vi "Edit Time Entry.vi"(8 "error in (no error)":errorcluster, 10 "Projects.lvclass":refnum<class "Projects.lvclass">, 11 "Time Entries in":refnum<class "Time Entries.lvclass">) -> (0 "error out":errorcluster, 3 "Time Entries out":refnum<class "Time Entries.lvclass">)   [LabVIEW 2020, in "Time Entries.lvclass"]
doc: "UI to edit the editable properties of the time entry.\n\n08/2025 Erich Schlieper"
uses:
  Time Entries.lvclass
  Projects/Parent/Projects.lvclass
  Time Entries.lvclass/Time Entries.ctl
panel:
  in  "Task":u16(ring)
  in  "Project":u16(ring)
  in  "End Time":timestamp format="%<%x %.3X>T"
  in  "Start Time":timestamp format="%<%x %.3X>T"
  in  "Description":string
  in  "Cancel":bool
  in  "OK":bool
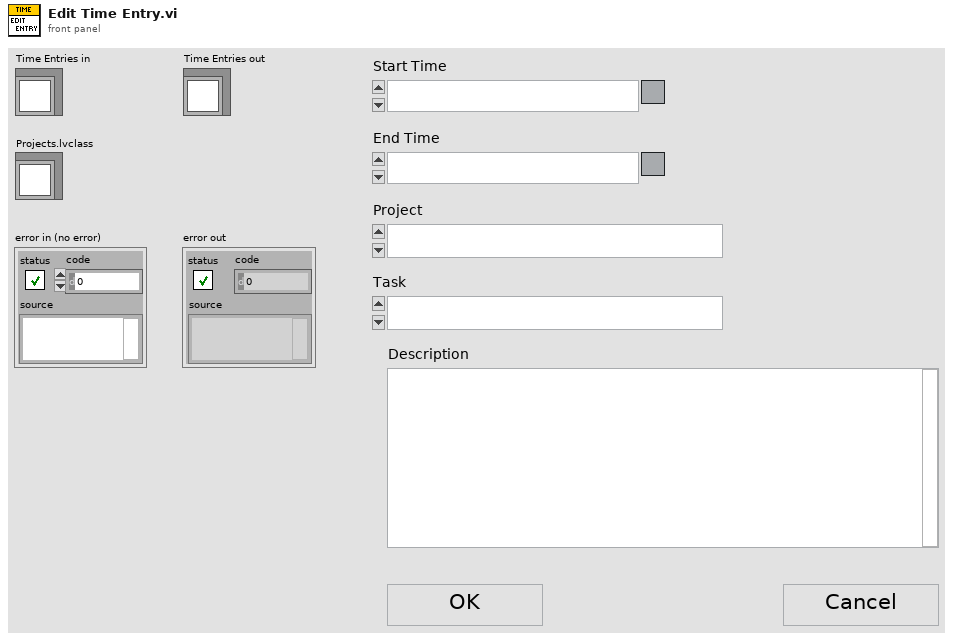
[diagram p1: front panel]
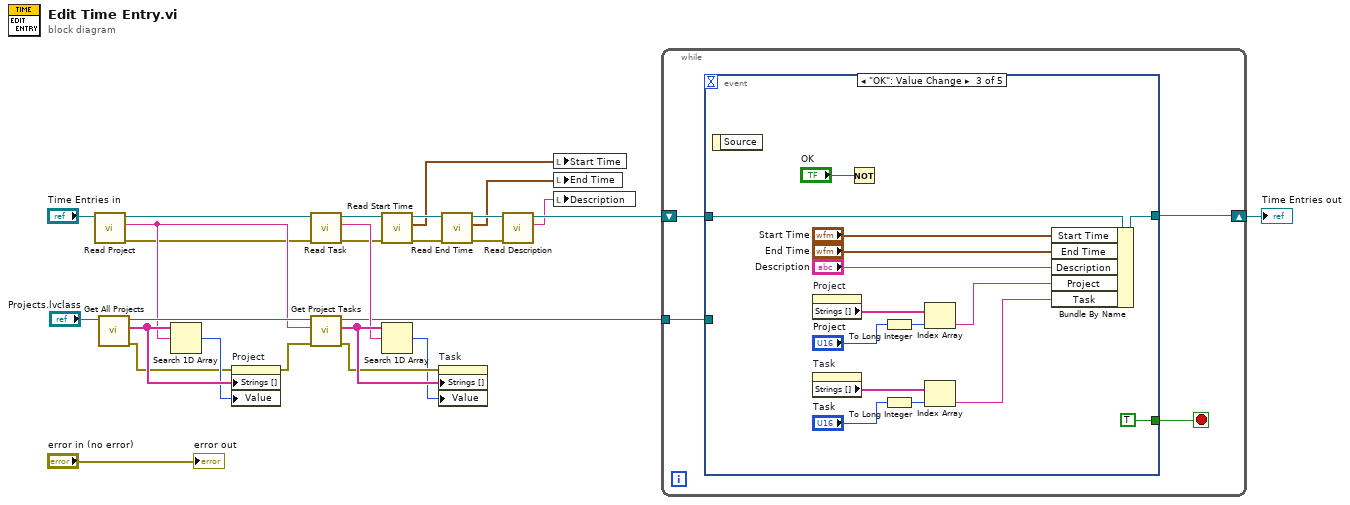
[diagram p0: block diagram]
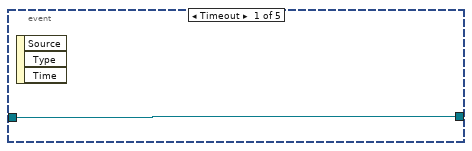
[diagram p2: hidden frame]
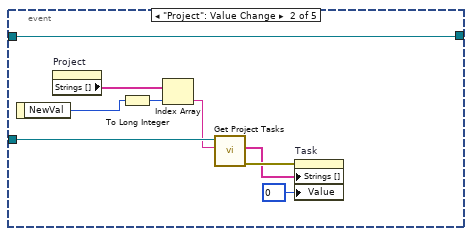
[diagram p3: hidden frame]
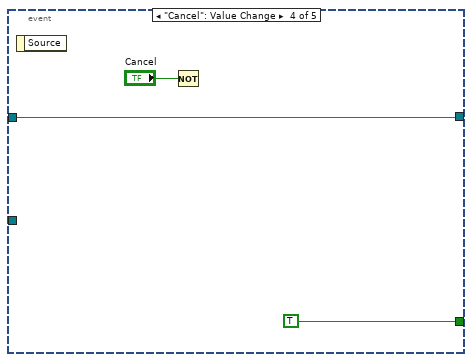
[diagram p4: hidden frame]
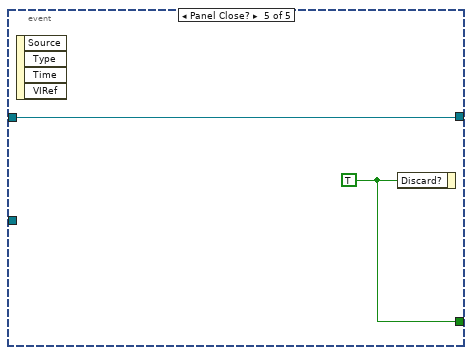
[diagram p5: hidden frame]
diagram:
  n1 = call-dynamic "Read Project.vi"("Time Entries in"="Time Entries in") -> ("error out"=w14:errorcluster, "Project"=w23:string, "Time Entries out"=w19:refnum<class "Time Entries.lvclass">)  [unwired: 8 in]
  n2 = call-dynamic "Get All Projects.vi"("Projects in"="Projects.lvclass") -> ("error out"=w21:errorcluster, "Projects"=w24:string[], "Projects out"=w25:refnum<class "Projects.lvclass">)  [unwired: 8 in]
  n3 = Search 1D Array(1D array=w24, element=w23) -> (index of element=w22:i32)  [unwired: 1 in]
  n4 = property on="Project" class="Ring (strict)"(error in=w21, "Strings []"=w24, "Value"=w22) -> (error out=w20:errorcluster)  [unwired: 1 in, 1 out]
  n5 = call-dynamic "Read Task.vi"("error in (no error)"=w14, "Time Entries in"=w19) -> ("error out"=w3:errorcluster, "Task"=w17:string, "Time Entries out"=w9:refnum<class "Time Entries.lvclass">)  [unwired: 7 in]
  n6 = call-dynamic "Get Project Tasks.vi"("error in (no error)"=w20, "Project Name"=w23, "Projects in"=w25) -> ("error out"=w16:errorcluster, "Tasks"=w18:string[], "Projects out"=w12:refnum<class "Projects.lvclass">)  [unwired: 6 in]
  n7 = call-dynamic "Read Start Time.vi"("error in (no error)"=w3, "Time Entries in"=w9) -> ("error out"=w2:errorcluster, "Start Time"=w7:timestamp, "Time Entries out"=w11:refnum<class "Time Entries.lvclass">)  [unwired: 7 in]
  n8 = Search 1D Array(1D array=w18, element=w17) -> (index of element=w15:i32)  [unwired: 1 in]
  n9 = property on="Task" class="Ring (strict)"(error in=w16, "Strings []"=w18, "Value"=w15) -> ()  [unwired: 1 in, 2 out]
  n10 = call-dynamic "Read End Time.vi"("error in (no error)"=w2, "Time Entries in"=w11) -> ("error out"=w1:errorcluster, "End Time"=w6:timestamp, "Time Entries out"=w10:refnum<class "Time Entries.lvclass">)  [unwired: 7 in]
  n11 = call-dynamic "Read Description.vi"("error in (no error)"=w1, "Time Entries in"=w10) -> ("Description"=w5:string, "Time Entries out"=w8:refnum<class "Time Entries.lvclass">)  [unwired: 7 in, 1 out]
  n12 = local write "Start Time"(w7) -> ()
  n13 = local write "End Time"(w6) -> ()
  n14 = local write "Description"(w5) -> ()
  n15 = while {
    shift-right: [w30] -> w13
    shift-left: w8 -> [w31]
    tunnel: w12 -> [w29]
    stop <- w28 stop-if-true
    n16 = event shown="[2] \"OK\": Value Change" {
      selector: _ -> [_ _ _ _ _]
      dyn-events: _ -> [_ _ _ _ _]
      timeout: _ -> [_ _ _ _ _]
      tunnel: w31 -> [w32 w35 w56 w59 w61]
      tunnel: [w32 w35 w54 w59 w61] -> w30
      tunnel: w29 -> [_ w39 _ _ _]
      tunnel: [_ _ TRUE TRUE w60] -> w28
      event Timeout {
        n17 = event-data() -> ()  [unwired: 1 in, 3 out]
      }
      event "Project": Value Change {
        w38 = u16 0 items=[""] ("Task")
        n18 = event-data() -> ("NewVal"=w33:u16)  [unwired: 1 in]
        n19 = property on="Project" class="Ring (strict)"() -> ("Strings []"=w37:string[])  [unwired: 2 in, 2 out]
        n20 = To Long Integer(number=w33) -> (32bit integer=w36:i32)
        n21 = Index Array(array=w37, index=w36) -> (element=w34:string)
        n22 = call-dynamic "Get Project Tasks.vi"("Project Name"=w34, "Projects in"=w39) -> ("error out"=w41:errorcluster, "Tasks"=w40:string[])  [unwired: 7 in, 1 out]
        n23 = property on="Task" class="Ring (strict)"(error in=w41, "Strings []"=w40, "Value"=w38) -> ()  [unwired: 1 in, 2 out]
      }
      event "OK": Value Change {
        n24 = event-data() -> ()  [unwired: 1 in, 1 out]
        n25 = property on="Project" class="Ring (strict)"() -> ("Strings []"=w48:string[])  [unwired: 2 in, 2 out]
        n26 = property on="Task" class="Ring (strict)"() -> ("Strings []"=w53:string[])  [unwired: 2 in, 2 out]
        n27 = Not(x="OK") -> ()  [unwired: 1 out]
        n28 = To Long Integer(number="Project") -> (32bit integer=w49:i32)
        n29 = To Long Integer(number="Task") -> (32bit integer=w52:i32)
        n30 = Index Array(array=w48, index=w49) -> (element=w44:string)
        n31 = Index Array(array=w53, index=w52) -> (element=w43:string)
        n32 = Bundle By Name(cluster=w56, "Start Time"="Start Time", "End Time"="End Time", "Description"="Description", "Project"=w44, "Task"=w43) -> (w54:refnum<class "Time Entries.lvclass">)
      }
      event "Cancel": Value Change {
        n33 = event-data() -> ()  [unwired: 1 in, 1 out]
        n34 = Not(x="Cancel") -> ()  [unwired: 1 out]
      }
      event Panel Close? {
        w60 = TRUE ("Discard?")
        n35 = event-data() -> ()  [unwired: 1 in, 4 out]
        n36 = event-data("Discard?"=w60) -> ()  [unwired: 1 in, 1 out]
      }
    }
  }
  "Time Entries out" <- w13
  "error out" <- "error in (no error)"
